vi "Read hostLoopPeriodAllowedJitter_percent.vi"(8 "error in (no error)":errorcluster, 11 "LoopConfig in":refnum<class "LoopConfig.lvclass">) -> (0 "error out":errorcluster, 2 "hostLoopPeriodAllowedJitter_percent":dbl=10.0, 3 "LoopConfig out":refnum<class "LoopConfig.lvclass">)   [LabVIEW 2013, in "ComponentData.lvlib" / "LoopConfig.lvclass"]
uses:
  <userlib>/Common/Component/Application/RT/ComponentData/ConfigurationHandler/LoopConfig/LoopConfig.lvclass
  <userlib>/Common/Component/Application/RT/ComponentData/ConfigurationHandler/LoopConfig/LoopConfig.lvclass/LoopConfig.ctl
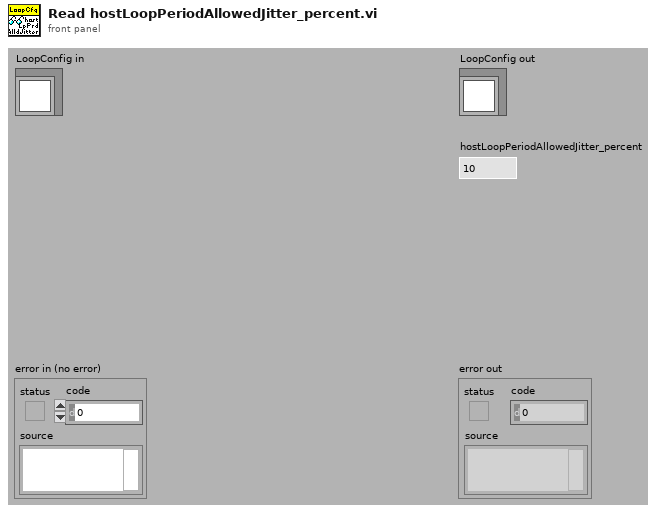
[diagram p1: front panel]
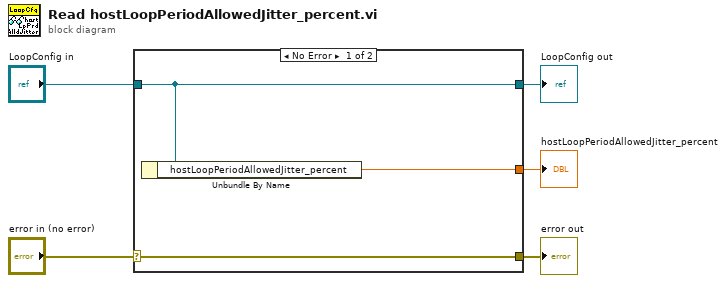
[diagram p0: block diagram]
diagram:
  n1 = case shown="No Error" "error in (no error)" {
    selector: "error in (no error)" -> [w8 w9]
    tunnel: [w8 w9] -> w4
    tunnel: [w7 w10] -> w2
    tunnel: "LoopConfig in" -> [w7 w10]
    tunnel: [w6 _] -> w1
    frame No Error {
      n2 = Unbundle By Name(w7) -> ("hostLoopPeriodAllowedJitter_percent"=w6:dbl)
    }
    frame Error {
    }
  }
  "error out" <- w4
  "LoopConfig out" <- w2
  "hostLoopPeriodAllowedJitter_percent" <- w1
